vi "Action.vi"(8 "b":dbl, 10 "a":dbl, 11 "add in":refnum<class "divide.lvclass">) -> (1 "result":dbl, 3 "add out":refnum<class "divide.lvclass">)   [LabVIEW 2020, in "divide.lvlib" / "divide.lvclass"]
uses:
  divide.lvclass
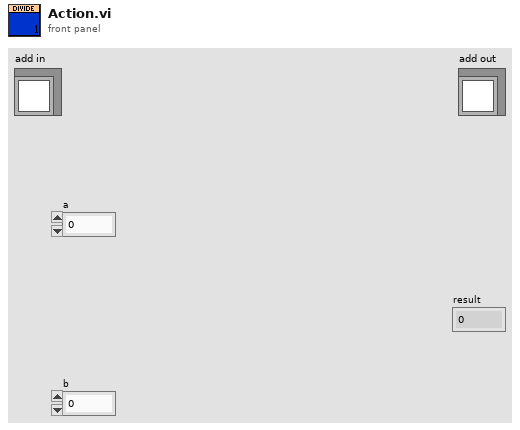
[diagram p1: front panel]
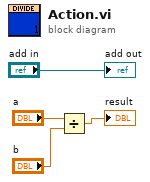
[diagram p0: block diagram]
diagram:
  n1 = Divide(x="a", y="b") -> (x/y=→"result":dbl)
  "add out" <- "add in"
